vi "Cypher Lithography 2.0_Feng.vi"(0 "Nodes on the line\n(  x      ,       y   )":dbl[][](array[numeric])=[[-5e-06, -5e-06], [5e-06, 5e-06]] min=-4.5e-05 max=4.5e-05 step=1e-09 format="%#_6pm", 1 "V":dbl[](array[numeric]), 2 "Litho Speed":dbl=5e-07 format="%#_6pm/s", 3 "Z SetPoint":dbl format="%#_6p", 4 "New nodes spacing":dbl=1e-06 format="%#_6pm", 5 "display wave":bool, 6 "Need interpolate new nodes?":bool, 7 "PID close":bool) -> ()   [LabVIEW 2013]
uses:
  <vilib>/Levylab/General AFM Lithography/subvi/Drivers/Cypher XY LVDT Parameters.vi
  <vilib>/Utility/file.llb/Write To Spreadsheet File (DBL).vi
panel:
  out "XY Graph":T1(graph)
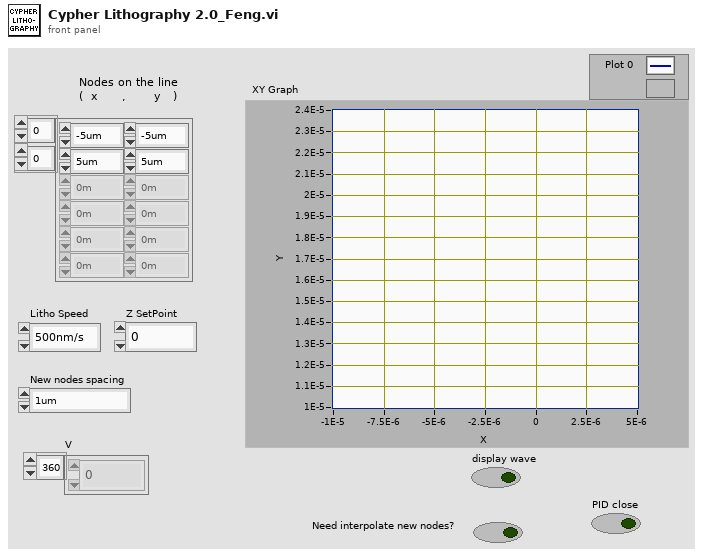
[diagram p1: front panel]
types:
  T1 = cluster{"Nodes on the line\n(  x      ,       y   )":dbl[], "Nodes on the line\n(  x      ,       y   )":dbl[]}[]
  T2 = cluster{"Interpolate result":dbl[], "Interpolate result":dbl[]}
  T3 = enum16{"open", "replace", "create", "open or create", "replace or create", "replace or create with confirmation"}
  T4 = cluster{"Nodes on the line\n(  x      ,       y   )":dbl[], "Nodes on the line\n(  x      ,       y   )":dbl[]}
  T5 = cluster{"Interpolate result":dbl[], "Interpolate result":dbl[]}[]
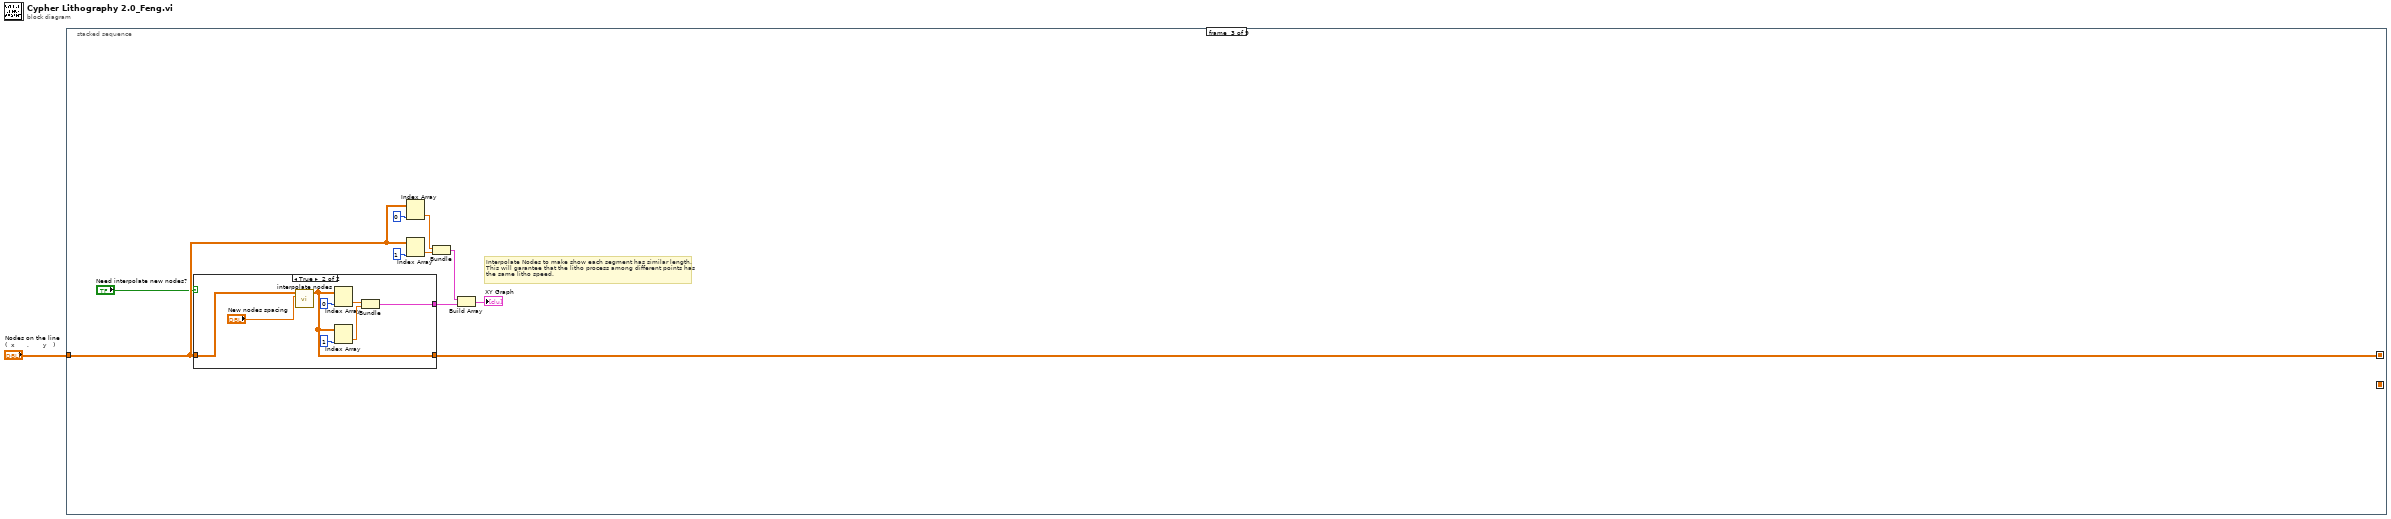
[diagram p0: block diagram]
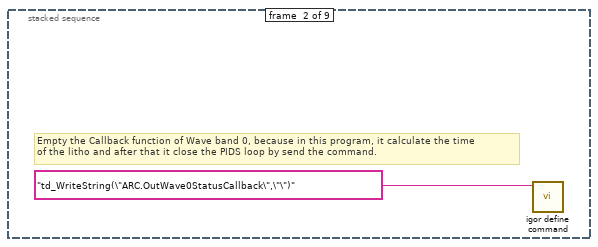
[diagram p3: hidden frame]
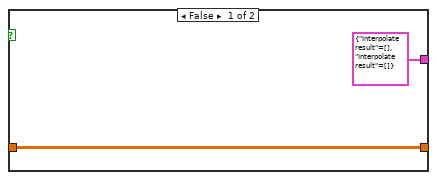
[diagram p4: hidden frame]
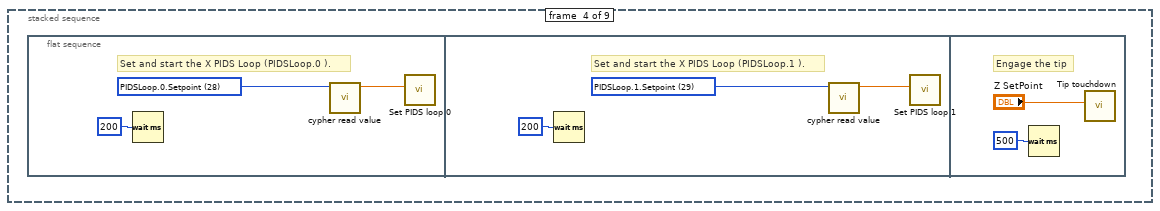
[diagram p5: hidden frame]
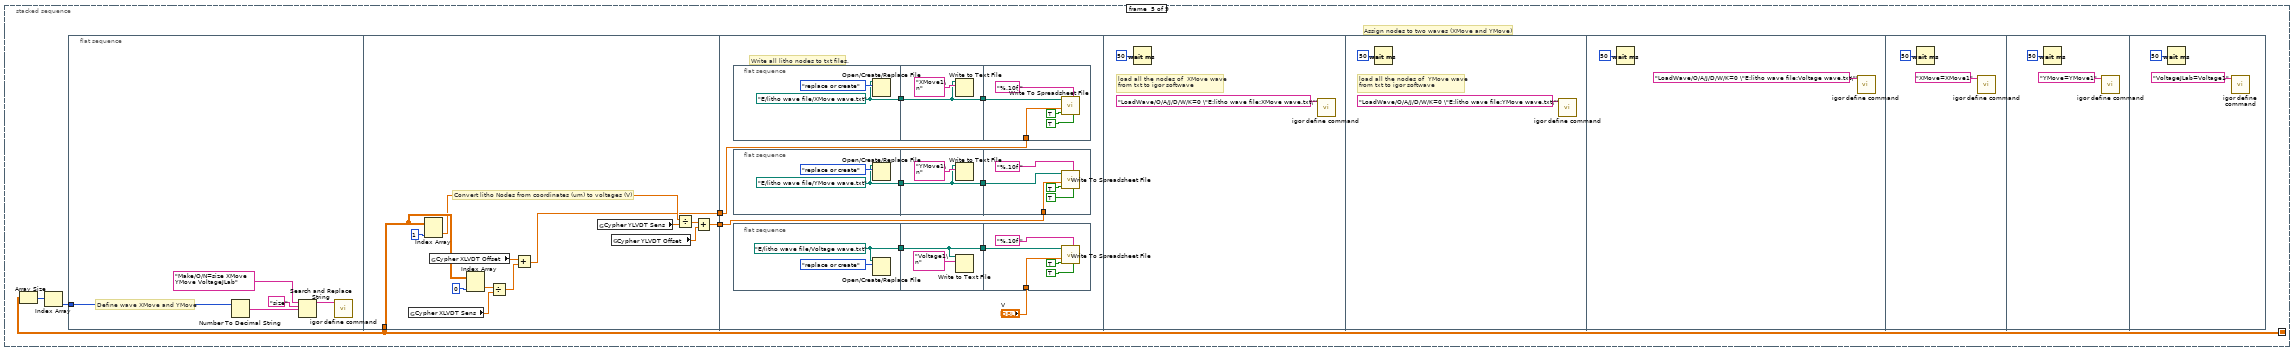
[diagram p6: hidden frame]
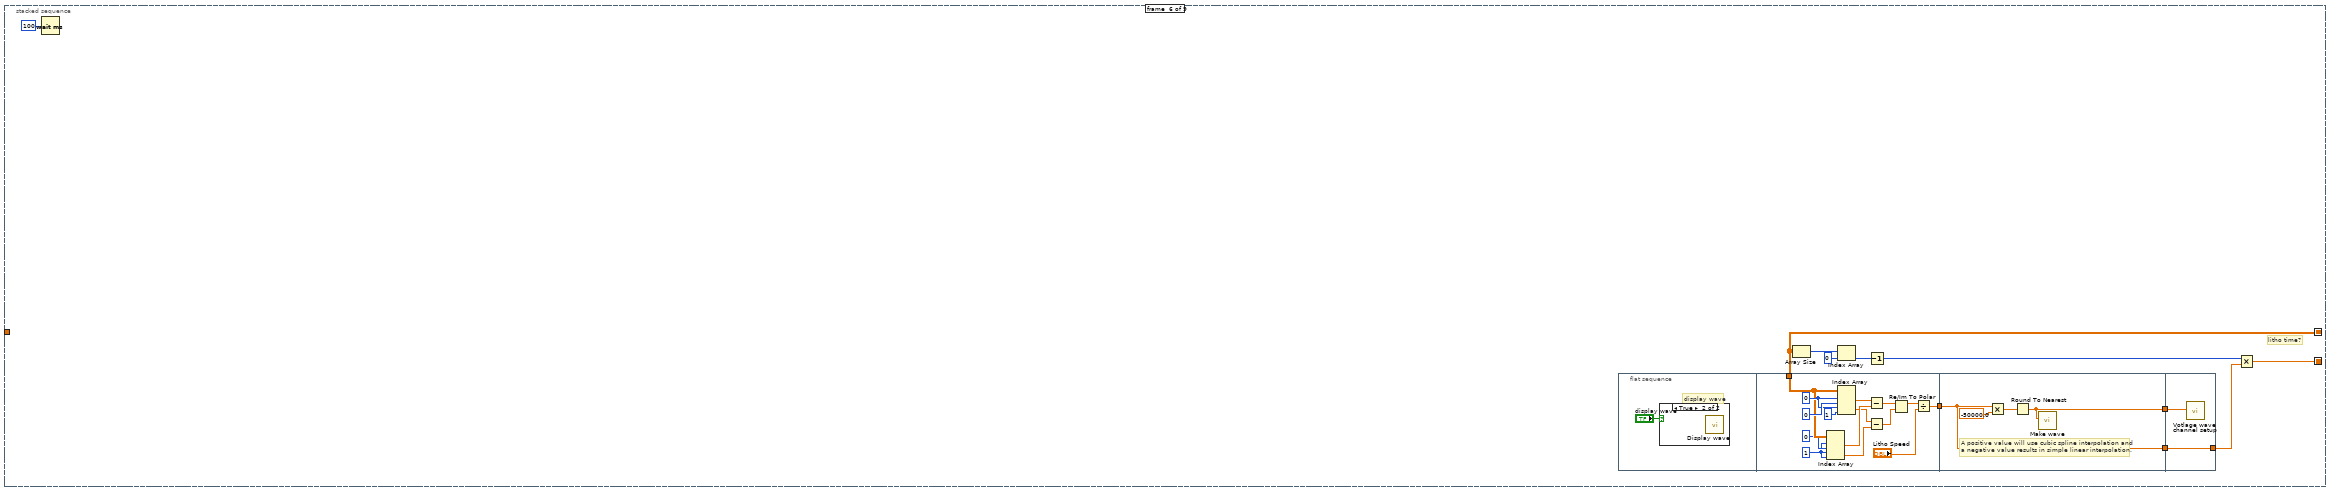
[diagram p7: hidden frame]
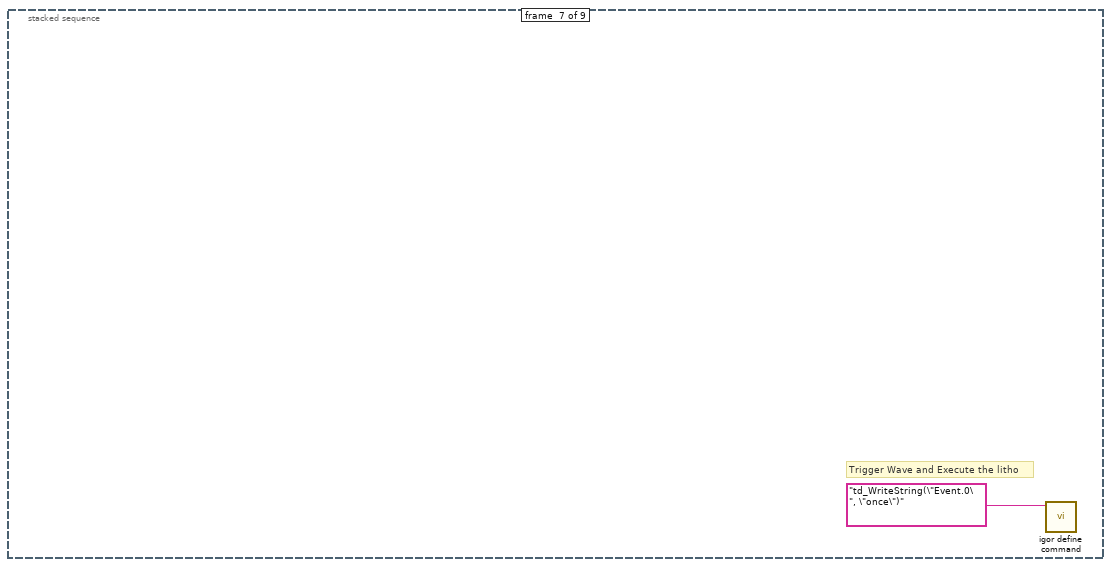
[diagram p9: hidden frame]
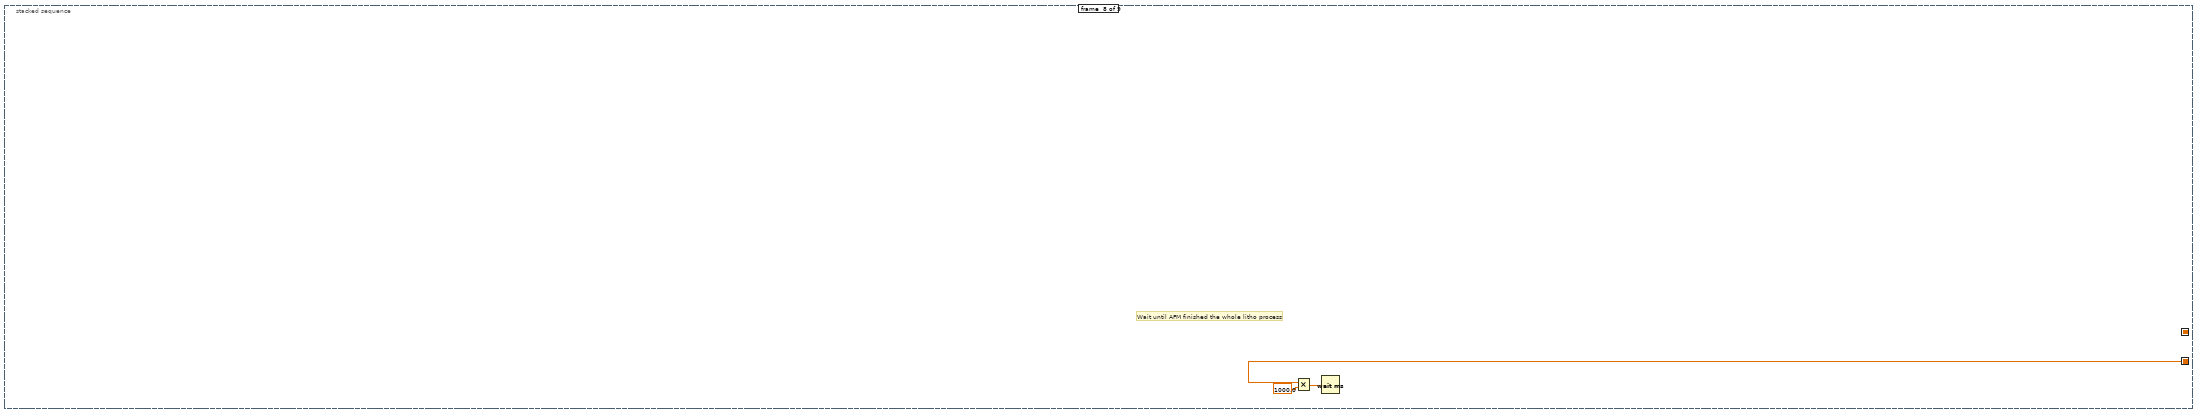
[diagram p10: hidden frame]
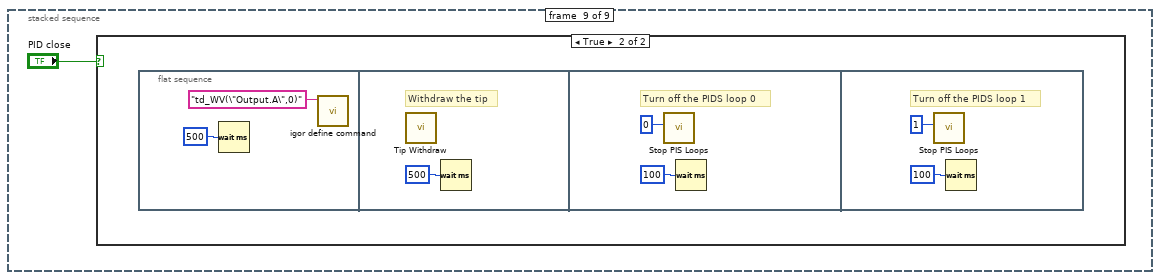
[diagram p11: hidden frame]
diagram:
  n1 = stacked-sequence {
    seq-local: [_ _ w4 _ _ _ _ _ _] -> [_ _ _ _ w32 w111 _ _ _]
    seq-local: [_ _ _ _ _ w107 _ _ _] -> [_ _ _ _ _ _ _ w138 _]
    tunnel: "Nodes on the line\n(  x      ,       y   )" -> [_ _ w6 _ _ _ _ _ _]
    frame #0 {
    }
    frame #1 {
      # "Empty the Callback function of Wave band 0, because in this program, it calculate the time \nof the litho and after that it close the PIDS loop by send the command."
      n2 = call "igor define command.vi"("Command"="td_WriteString(\"ARC.OutWave0StatusCallback\",\"\")") -> ()  [unwired: 11 out]
    }
    frame #2 {
      # "Interpolate Nodes to make show each segment has similar length.\nThis will garantee that the litho process among different points has\nthe same litho speed."
      n3 = case shown="True" "Need interpolate new nodes?" {
        tunnel: w6 -> [w14 w22]
        tunnel: [T2 {"Interpolate result"=[], "Interpolate result"=[]} w17] -> w5
        tunnel: [w14 w16] -> w4
        frame False {
        }
        frame True {
          n4 = call "interpolate nodes.vi"("Interpolate spacing"="New nodes spacing", "Nodes on the line\n(  x      ,       y   )"=w22) -> ("Interpolate result"=w16:dbl[][])  [unwired: 9 in]
          n5 = Index Array(array=w16, index (col)=0 ("disabled index (col)")) -> (element=w19:dbl[])  [unwired: 1 in]
          n6 = Index Array(array=w16, index (col)=1 ("disabled index (col)")) -> (element=w18:dbl[])  [unwired: 1 in]
          n7 = Bundle("Interpolate result"=w19, "Interpolate result"=w18) -> (w17:T2)  [unwired: 1 in]
        }
      }
      n8 = Index Array(array=w6, index (col)=0 ("disabled index (col)")) -> (element=w11:dbl[])  [unwired: 1 in]
      n9 = Index Array(array=w6, index (col)=1 ("disabled index (col)")) -> (element=w9:dbl[])  [unwired: 1 in]
      n10 = Bundle("Nodes on the line\n(  x      ,       y   )"=w11, "Nodes on the line\n(  x      ,       y   )"=w9) -> (w8:T4)  [unwired: 1 in]
      n11 = Build Array(w8, w5) -> (→"XY Graph":T5)
    }
    frame #3 {
      n12 = flat-sequence {
        frame #0 {
          w24 = u16 28 items=["XSensor", "YSensor", "ZSensor", "InA", "InB", "InFast", "In_Amplitude1", "In_Amplitude2", "In_Phase1", "In_Phase2", "PiezoX", "PiezoY", "PiezoZ", "OutA", "OutB", "OutC", "DDS_Frequency1", "DDS_Frequency2", "DDS_Amplitude1", "DDS_Amplitude2", "DDS_DCOffset", "Laser_Sum", "Laser_Difference", "Laser_Lateral", "XLVDT Sensitivity", "YLVDT Sensitivity", "XLVDT Offset", "YLVDT Offset", "PIDSLoop.0.Setpoint", "PIDSLoop.1.Setpoint"] ("Input")
          # "Set and start the X PIDS Loop (PIDSLoop.0 )."
          n13 = Wait (ms)(milliseconds to wait=u32 200) -> ()  [unwired: 1 out]
          n14 = call "cypher read value.vi"("Input"=w24) -> ("Result"=w25:dbl)  [unwired: 10 in]
          n15 = call "Set PIDS loop 0.vi"("X  Setpoint"=w25) -> ()  [unwired: 11 in]
        }
        frame #1 {
          w27 = u16 29 items=["XSensor", "YSensor", "ZSensor", "InA", "InB", "InFast", "In_Amplitude1", "In_Amplitude2", "In_Phase1", "In_Phase2", "PiezoX", "PiezoY", "PiezoZ", "OutA", "OutB", "OutC", "DDS_Frequency1", "DDS_Frequency2", "DDS_Amplitude1", "DDS_Amplitude2", "DDS_DCOffset", "Laser_Sum", "Laser_Difference", "Laser_Lateral", "XLVDT Sensitivity", "YLVDT Sensitivity", "XLVDT Offset", "YLVDT Offset", "PIDSLoop.0.Setpoint", "PIDSLoop.1.Setpoint"] ("Input")
          # "Set and start the X PIDS Loop (PIDSLoop.1 )."
          n16 = Wait (ms)(milliseconds to wait=u32 200) -> ()  [unwired: 1 out]
          n17 = call "cypher read value.vi"("Input"=w27) -> ("Result"=w28:dbl)  [unwired: 10 in]
          n18 = call "Set PIDS loop 1.vi"("Y Setpoint"=w28) -> ()  [unwired: 11 in]
        }
        frame #2 {
          # "Engage the tip"
          n19 = Wait (ms)(milliseconds to wait=u32 500) -> ()  [unwired: 1 out]
          n20 = call "Tip touchdown.vi"("Z SetPoint"="Z SetPoint") -> ()  [unwired: 11 out]
        }
      }
    }
    frame #4 {
      # "Assign nodes to two waves (XMove and YMove)"
      n21 = Array Size(array=w32) -> (size(s)=w33:i32[])
      n22 = Index Array(array=w33) -> (element=w31:i32)  [unwired: 1 in]
      n23 = flat-sequence {
        tunnel: w31 -> [w36]
        tunnel: w32 -> [w46]
        tunnel: [w42] -> w35
        tunnel: [w41] -> w34
        tunnel: w35 -> [w58]
        tunnel: w34 -> [w57]
        frame #0 {
          # "Define wave XMove and YMove"
          n24 = Number To Decimal String(number=w36) -> (decimal integer string=w38:string)  [unwired: 1 in]
          n25 = Search and Replace String(input string="Make/O/N=size XMove YMove VoltageJLab", search string="size", replace string=w38) -> (result string=w37:string)  [unwired: 1 in, 7 out]
          n26 = call "igor define command.vi"("Command"=w37) -> ()  [unwired: 11 out]
        }
        frame #1 {
          # "Convert litho Nodes from coordinates (um) to voltages (V)"
          n27 = global read "Cypher XY LVDT Parameters.vi" "Cypher XLVDT Sens"() -> (w49:dbl)
          n28 = Index Array(array=w46, index (col)=1 ("disabled index (col)")) -> (element=w43:dbl[])  [unwired: 1 in]
          n29 = global read "Cypher XY LVDT Parameters.vi" "Cypher XLVDT Offset"() -> (w48:dbl)
          n30 = Index Array(array=w46, index (col)=0 ("disabled index (col)")) -> (element=w44:dbl[])  [unwired: 1 in]
          n31 = Divide(x=w44, y=w49) -> (x/y=w52:dbl[])
          n32 = Add(x=w48, y=w52) -> (x+y=w41:dbl[])
          n33 = global read "Cypher XY LVDT Parameters.vi" "Cypher YLVDT Sens"() -> (w50:dbl)
          n34 = global read "Cypher XY LVDT Parameters.vi" "Cypher YLVDT Offset"() -> (w47:dbl)
          n35 = Divide(x=w43, y=w50) -> (x/y=w51:dbl[])
          n36 = Add(x=w51, y=w47) -> (x+y=w42:dbl[])
        }
        frame #2 {
          # "Write all litho nodes to txt files."
          n37 = flat-sequence {
            tunnel: [w81] -> w62
            tunnel: w62 -> [w83]
            tunnel: [w83] -> w61
            tunnel: w61 -> [w87]
            tunnel: w57 -> [w86]
            frame #0 {
              w81 = path "E:/litho wave file/XMove wave.txt" ("\"XMove wave\" file path")
              n38 = Open/Create/Replace File(file path (use dialog)=w81, operation (0:open)=T3."replace or create") -> ()  [unwired: 4 in, 3 out]
            }
            frame #1 {
              n39 = Write to Text File(file (use dialog)=w83, text="XMove1\n") -> ()  [unwired: 2 in, 3 out]
            }
            frame #2 {
              n40 = call-poly <vilib>:"Write To Spreadsheet File.vi"("transpose? (no:F)"=TRUE, "format (%.3f)"="%.10f ", "append to file? (new file:F)"=TRUE, "1D data"=w86, "file path (dialog if empty)"=w87) -> ()  [unwired: 3 in, 1 out]
            }
          }
          n41 = flat-sequence {
            tunnel: [w72] -> w60
            tunnel: w60 -> [w74]
            tunnel: [w74] -> w59
            tunnel: w59 -> [w78]
            tunnel: w58 -> [w77]
            frame #0 {
              w72 = path "E:/litho wave file/YMove wave.txt" ("\"YMove wave\" file path")
              n42 = Open/Create/Replace File(file path (use dialog)=w72, operation (0:open)=T3."replace or create") -> ()  [unwired: 4 in, 3 out]
            }
            frame #1 {
              n43 = Write to Text File(file (use dialog)=w74, text="YMove1\n") -> ()  [unwired: 2 in, 3 out]
            }
            frame #2 {
              n44 = call-poly <vilib>:"Write To Spreadsheet File.vi"("transpose? (no:F)"=TRUE, "format (%.3f)"="%.10f ", "append to file? (new file:F)"=TRUE, "1D data"=w77, "file path (dialog if empty)"=w78) -> ()  [unwired: 3 in, 1 out]
            }
          }
          n45 = flat-sequence {
            tunnel: [w63] -> w56
            tunnel: w56 -> [w65]
            tunnel: [w65] -> w55
            tunnel: w55 -> [w69]
            tunnel: "V" -> [w67]
            frame #0 {
              w63 = path "E:/litho wave file/Voltage wave.txt" ("file path (use dialog)")
              n46 = Open/Create/Replace File(file path (use dialog)=w63, operation (0:open)=T3."replace or create") -> ()  [unwired: 4 in, 3 out]
            }
            frame #1 {
              n47 = Write to Text File(file (use dialog)=w65, text="Voltage1\n") -> ()  [unwired: 2 in, 3 out]
            }
            frame #2 {
              n48 = call-poly <vilib>:"Write To Spreadsheet File.vi"("transpose? (no:F)"=TRUE, "format (%.3f)"="%.10f ", "append to file? (new file:F)"=TRUE, "1D data"=w67, "file path (dialog if empty)"=w69) -> ()  [unwired: 3 in, 1 out]
            }
          }
        }
        frame #3 {
          # "load all the nodes of  XMove wave\nfrom txt to igor softwave"
          n49 = Wait (ms)(milliseconds to wait=u32 50) -> ()  [unwired: 1 out]
          n50 = call "igor define command.vi"("Command"="LoadWave/O/A/J/D/W/K=0 \"E:litho wave file:XMove wave.txt\"") -> ()  [unwired: 11 out]
        }
        frame #4 {
          # "load all the nodes of  YMove wave\nfrom txt to igor softwave"
          n51 = Wait (ms)(milliseconds to wait=u32 50) -> ()  [unwired: 1 out]
          n52 = call "igor define command.vi"("Command"="LoadWave/O/A/J/D/W/K=0 \"E:litho wave file:YMove wave.txt\"") -> ()  [unwired: 11 out]
        }
        frame #5 {
          n53 = Wait (ms)(milliseconds to wait=u32 50) -> ()  [unwired: 1 out]
          n54 = call "igor define command.vi"("Command"="LoadWave/O/A/J/D/W/K=0 \"E:litho wave file:Voltage wave.txt\"") -> ()  [unwired: 11 out]
        }
        frame #6 {
          n55 = Wait (ms)(milliseconds to wait=u32 50) -> ()  [unwired: 1 out]
          n56 = call "igor define command.vi"("Command"="XMove=XMove1") -> ()  [unwired: 11 out]
        }
        frame #7 {
          n57 = Wait (ms)(milliseconds to wait=u32 50) -> ()  [unwired: 1 out]
          n58 = call "igor define command.vi"("Command"="YMove=YMove1") -> ()  [unwired: 11 out]
        }
        frame #8 {
          n59 = Wait (ms)(milliseconds to wait=u32 50) -> ()  [unwired: 1 out]
          n60 = call "igor define command.vi"("Command"="VoltageJLab=Voltage1") -> ()  [unwired: 11 out]
        }
      }
    }
    frame #5 {
      # "litho time?"
      n61 = Wait (ms)(milliseconds to wait=u32 100) -> ()  [unwired: 1 out]
      n62 = flat-sequence {
        tunnel: w111 -> [w125]
        tunnel: [w114] -> w112
        tunnel: w112 -> [w130]
        tunnel: [w130] -> w103
        tunnel: [w129] -> w102
        tunnel: [w134] -> w108
        tunnel: w103 -> [w134]
        tunnel: w102 -> [w133]
        frame #0 {
          # "display wave"
          n63 = case shown="True" "display wave" {
            frame False {
            }
            frame True {
              n64 = call "Display wave.vi"() -> ()  [unwired: 1 out]
            }
          }
        }
        frame #1 {
          w123 = 1 ("index (row)")
          w127 = 0 ("index (row)")
          n65 = Index Array(array=w125, index (row) #1=w123, index (col) #1=0 ("disabled index (col)"), index (row) #2=w123, index (col) #2=w123) -> (element #1=w121:dbl, element #2=w120:dbl)
          n66 = Index Array(array=w125, index (row) #1=w127, index (col) #1=0 ("disabled index (col)"), index (row) #2=w127, index (col) #2=1 ("disabled index (col)")) -> (element #1=w122:dbl, element #2=w119:dbl)
          n67 = Subtract(x=w122, y=w121) -> (x-y=w118:dbl)
          n68 = Subtract(x=w119, y=w120) -> (x-y=w117:dbl)
          n69 = Re/Im To Polar(2:w117, 3:w118) -> (1:w116:dbl)  [unwired: 1 out]
          n70 = Divide(x=w116, y="Litho Speed") -> (x/y=w114:dbl)
        }
        frame #2 {
          # "A positive value will use cubic spline interpolation and \na negative value results in simple linear interpolation."
          n71 = Multiply(x=w130, y=-50000.0) -> (x*y=w131:dbl)
          n72 = Round To Nearest(number=w131) -> (nearest integer value=w129:dbl)
          n73 = call "Make wave.vi"("Totalpoints"=w129) -> ()  [unwired: 11 out]
        }
        frame #3 {
          n74 = call "Votlage wave channel setup.vi"("Totalpoints"=w133) -> ()  [unwired: 11 in]
        }
      }
      n75 = Array Size(array=w111) -> (size(s)=w110:i32[])
      n76 = Index Array(array=w110, index=0) -> (element=w106:i32)
      n77 = Decrement(x=w106) -> (x-1=w105:i32)
      n78 = Multiply(x=w105, y=w108) -> (x*y=w107:dbl)
    }
    frame #6 {
      # "Trigger Wave and Execute the litho"
      n79 = call "igor define command.vi"("Command"="td_WriteString(\"Event.0\", \"once\")") -> ()  [unwired: 11 out]
    }
    frame #7 {
      # "Wait until AFM finished the whole litho process"
      n80 = Multiply(x=w138, y=1000.0) -> (x*y=w136:dbl)
      n81 = Wait (ms)(milliseconds to wait=w136) -> ()  [unwired: 1 out]
    }
    frame #8 {
      n82 = case shown="True" "PID close" {
        frame False {
        }
        frame True {
          n83 = flat-sequence {
            frame #0 {
              n84 = Wait (ms)(milliseconds to wait=u32 500) -> ()  [unwired: 1 out]
              n85 = call "igor define command.vi"("Command"="td_WV(\"Output.A\",0)") -> ()  [unwired: 11 out]
            }
            frame #1 {
              # "Withdraw the tip"
              n86 = call "Tip Withdraw.vi"() -> ()  [unwired: 1 in]
              n87 = Wait (ms)(milliseconds to wait=u32 500) -> ()  [unwired: 1 out]
            }
            frame #2 {
              # "Turn off the PIDS loop 0"
              n88 = call "Stop PIS Loops.vi"("PIS Loop Number (0-5)"=u32 0) -> ()  [unwired: 11 out]
              n89 = Wait (ms)(milliseconds to wait=u32 100) -> ()  [unwired: 1 out]
            }
            frame #3 {
              # "Turn off the PIDS loop 1"
              n90 = call "Stop PIS Loops.vi"("PIS Loop Number (0-5)"=u32 1) -> ()  [unwired: 11 out]
              n91 = Wait (ms)(milliseconds to wait=u32 100) -> ()  [unwired: 1 out]
            }
          }
        }
      }
    }
  }
